vi "Calculate Result Values.vi"(8 "error in":errorcluster, 10 "Signals in":waveform(dbl)[](array[waveform]), 11 "DAC Keller BNC in":refnum<class "DAC Keller BNC.lvclass">) -> (0 "error out":errorcluster, 2 "Signals out":waveform(dbl)[](array[waveform]), 3 "DAC Keller BNC out":refnum<class "DAC Keller BNC.lvclass">)   [LabVIEW 2019, in "DAC.lvlib" / "DAC Keller BNC.lvclass"]
uses:
  DAC Keller BNC.lvclass
  DAC Keller BNC.lvclass/DAC Keller BNC.ctl
  <vilib>/measure/madcrms.llb/Basic Averaged DC-RMS for 1 Chan.vi
  <vilib>/measure/NI_MAPro.lvlib
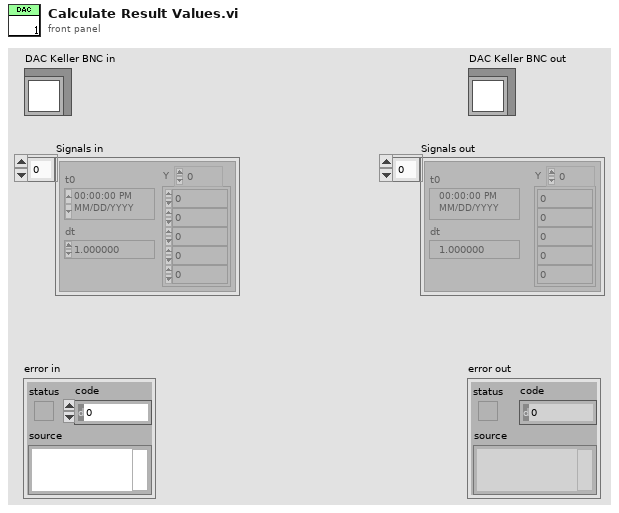
[diagram p1: front panel]
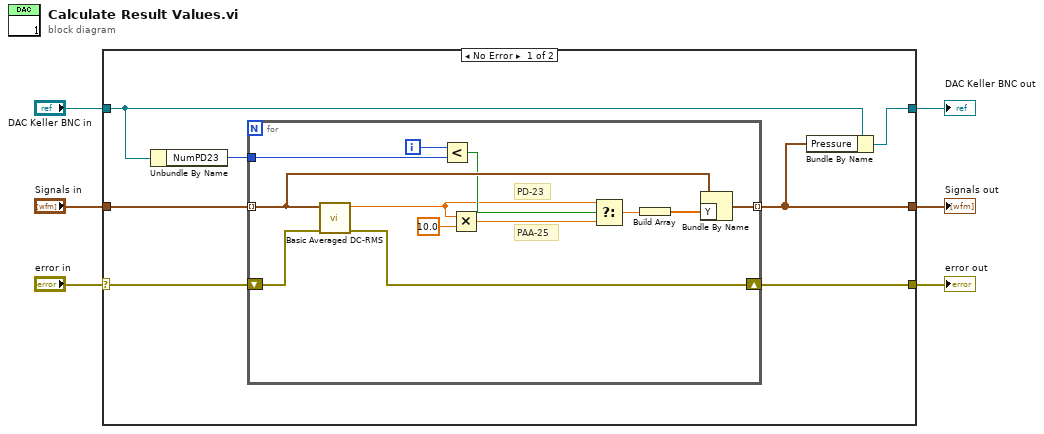
[diagram p0: block diagram]
diagram:
  n1 = case shown="No Error" "error in" {
    selector: "error in" -> [w10 w28]
    tunnel: [w9 w28] -> w5
    tunnel: [w13 w27] -> w3
    tunnel: "DAC Keller BNC in" -> [w8 w27]
    tunnel: "Signals in" -> [w12 w26]
    tunnel: [w11 w26] -> w1
    frame No Error {
      n2 = Unbundle By Name(w8) -> ("NumPD23"=w7:i32)
      n3 = for {
        tunnel: w12 -> [w24] mode=indexing
        tunnel: [w23] -> w11 mode=indexing
        shift-right: [w21] -> w9
        shift-left: w10 -> [w22]
        tunnel: w7 -> [w19]
        i -> [w20]
        # "PAA-25"
        # "PD-23"
        n4 = call-poly <vilib>:"Basic Averaged DC-RMS.vi"("error in (no error)"=w22, "signal in"=w24) -> ("error out"=w21:errorcluster, "DC value"=w17:dbl)  [unwired: 6 in, 2 out]
        n5 = Less?(x=w20, y=w19) -> (x < y?=w18:bool)
        n6 = Multiply(x=w17, y=10.0) -> (x*y=w15:dbl)
        n7 = Select(t=w17, s=w18, f=w15) -> (s? t:f=w14:dbl)
        n8 = Build Array(w14) -> (w25:dbl[])
        n9 = Bundle By Name(cluster=w24, "Y"=w25) -> (w23:waveform(dbl))
      }
      n10 = Bundle By Name(cluster=w8, "Pressure"=w11) -> (w13:refnum<class "DAC Keller BNC.lvclass">)
    }
    frame Error {
    }
  }
  "error out" <- w5
  "DAC Keller BNC out" <- w3
  "Signals out" <- w1
